vi "Protocol Write.vi"(8 "error in (no error)":errorcluster, 9 "timeout":i32=10000, 10 "data":u8[](array[numeric]), 11 "protocol layer in":refnum<class "Serial Master.lvclass">) -> (0 "error out":errorcluster, 1 "timed out?":bool, 3 "protocol layer out":refnum<class "Serial Master.lvclass">)   [LabVIEW 2018, in "SubVIs.lvlib" / "Serial Master.lvclass"]
doc: "This provides an interface for writing to a network bus."
uses:
  Serial Master.lvclass
  Serial Master.lvclass/Serial Master.ctl
  Serial Shared Components.lvlib
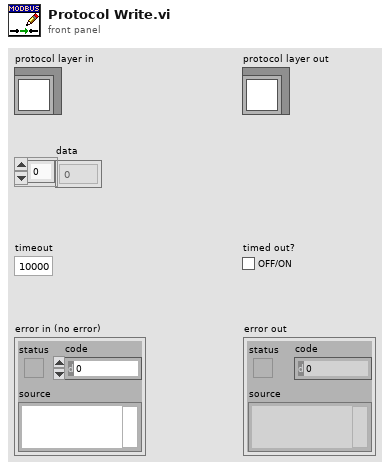
[diagram p1: front panel]
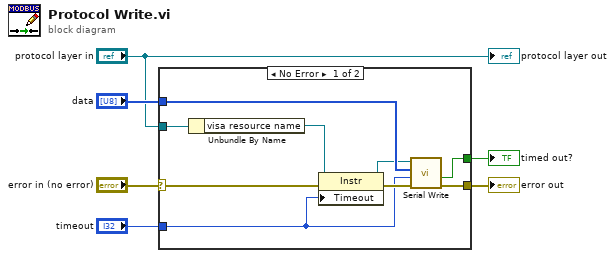
[diagram p0: block diagram]
diagram:
  n1 = case shown="No Error" "error in (no error)" {
    selector: "error in (no error)" -> [w11 w16]
    tunnel: [w15 w16] -> w6
    tunnel: [w14 _] -> w5
    tunnel: "timeout" -> [w7 _]
    tunnel: "data" -> [w13 _]
    tunnel: "protocol layer in" -> [w12 _]
    frame No Error {
      n2 = Unbundle By Name(w12) -> ("visa resource name"=w9:refnum<visa-resource-name>)
      n3 = property class="Instr"(reference=w9, error in=w11, "Timeout"=w7) -> (reference out=w8:refnum<visa-resource-name>, error out=w10:errorcluster)
      n4 = call "Serial Write.vi"("error in (no error)"=w10, "timeout (ms)"=w7, "data"=w13, "VISA resource"=w8) -> ("error out"=w15:errorcluster, "timed out?"=w14:bool)  [unwired: 6 in]
    }
    frame Error {
    }
  }
  "error out" <- w6
  "timed out?" <- w5
  "protocol layer out" <- "protocol layer in"
